vi "Prepare Controls Refs.vi"(9 "Numeric":i32, 10 "Controls[]":refnum<vi>[](array[refnum]), 11 "Boolean in":refnum<vi>) -> (3 "Boolean out":refnum<vi>)   [LabVIEW 2019]
doc: "Get Controlled element (LED) by indexing and then typecast to boolean."
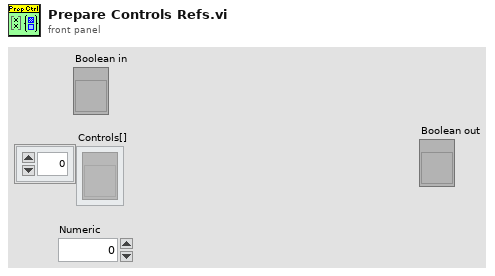
[diagram p1: front panel]
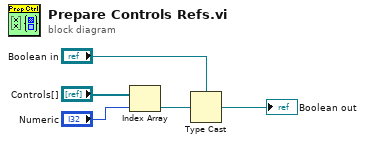
[diagram p0: block diagram]
diagram:
  n1 = Index Array(array="Controls[]", index="Numeric") -> (element=w3:refnum<vi>)
  n2 = Type Cast(type="Boolean in", x=w3) -> (*(type *) &x=→"Boolean out":refnum<vi>)
